vi "Search Strings.vi"() -> ()   [LabVIEW 2011]
uses:
  Modules/Hardware/Mass Flow Controller/Valve Status.ctl
  Modules/Hardware/Mass Flow Controller/Mass Flow Controller.lvclass
panel:
  out "after substring":string
  in  "Valve Status":T1
  out "resulting string":string
  out "Status Bar String OUT":string
  in  "Status Bar String IN":string="MFC = 200ml/min; PS =30V"
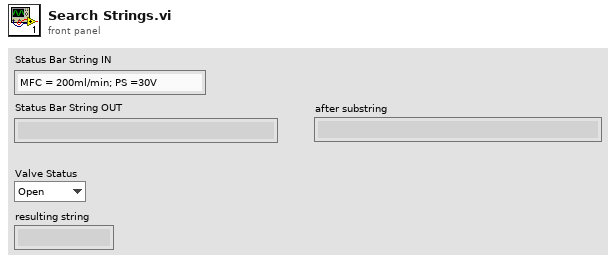
[diagram p1: front panel]
types:
  T1 = typedef "Mass Flow Controller.lvclass/Valve Status.ctl" = enum16{"Open", "Closed"}
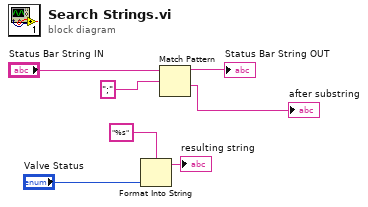
[diagram p0: block diagram]
diagram:
  n1 = Format Into String(format string="%s", "Valve Status") -> (resulting string=→"resulting string":string)  [unwired: 2 in, 1 out]
  n2 = Match Pattern(string="Status Bar String IN", regular expression=";") -> (before substring=→"Status Bar String OUT":string, after substring=→"after substring":string)  [unwired: 1 in, 2 out]
